vi "Configure Receiver Information.vi"(5 "Receiver (0: R1)":u16(ring) items=["R1", "R2", "A", "B"], 6 "Power Offset (0)":dbl, 7 "Enable Receiver Correction (F: Disabled)":bool, 8 "error in (no error)":errorcluster, 9 "Port (1)":i32=1, 10 "Channel (1)":i32=1, 11 "VISA resource name":refnum<visa-resource-name>) -> (0 "error out":errorcluster, 3 "VISA resource name out":refnum<visa-resource-name>)   [LabVIEW 2022 SP3, in "Agilent ENA Series.lvlib"]
doc: "Configures information for the receiver R1, R2, A, or B.\n\nNote:\nValid for E5072A only."
uses:
  <instrlib>/Agilent ENA Series/Agilent ENA Series.lvlib
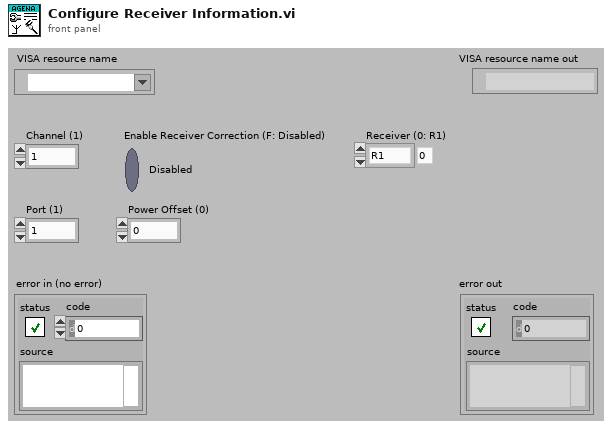
[diagram p1: front panel]
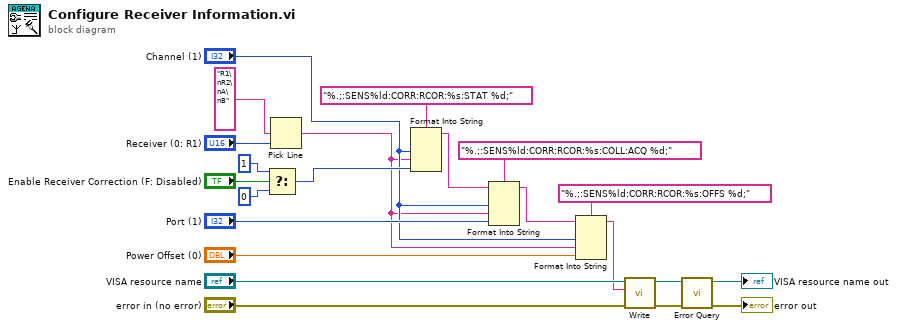
[diagram p0: block diagram]
diagram:
  n1 = Select(t=1, s="Enable Receiver Correction (F: Disabled)", f=0) -> (s? t:f=w10:i32)
  n2 = Pick Line(multi-line string="R1\nR2\nA\nB", line index="Receiver (0: R1)") -> (output string=w5:string)  [unwired: 1 in]
  n3 = Format Into String(format string="%.;:SENS%ld:CORR:RCOR:%s:STAT %d;", "Channel (1)", w5, w10) -> (resulting string=w1:string)  [unwired: 2 in, 1 out]
  n4 = Format Into String(format string="%.;:SENS%ld:CORR:RCOR:%s:COLL:ACQ %d;", initial string=w1, "Channel (1)", w5, "Port (1)") -> (resulting string=w2:string)  [unwired: 1 in, 1 out]
  n5 = Format Into String(format string="%.;:SENS%ld:CORR:RCOR:%s:OFFS %d;", initial string=w2, "Channel (1)", w5, "Power Offset (0)") -> (resulting string=w3:string)  [unwired: 1 in, 1 out]
  n6 = call <instrlib>:"Write.vi"("error in (no error)"="error in (no error)", "String ()"=w3, "VISA resource name"="VISA resource name") -> ("error out"=w22:errorcluster, "VISA resource name out"=w21:refnum<visa-resource-name>)  [unwired: 6 in, 1 out]
  n7 = call <instrlib>:"Error Query.vi"("error in (no error)"=w22, "VISA resource name"=w21) -> ("error out"=→"error out":errorcluster, "VISA resource name out"=→"VISA resource name out":refnum<visa-resource-name>)  [unwired: 6 in, 2 out]
